vi "PCI-USB_ Untitled 1.vi"() -> ()   [LabVIEW 2015]
panel:
  in  "Output":T1={"DO"=FALSE, "DO 2"=FALSE, "DO 3"=FALSE, "DO 4"=FALSE, "DO 5"=FALSE, "DO 6"=FALSE, "DO 7"=FALSE, "DO 8"=FALSE, "DO 9"=FALSE, "DO 10"=FALSE, "DO 11"=FALSE, "DO 12"=FALSE, "DO 13"=FALSE, "DO 14"=FALSE, "DO 15"=FALSE, "DO 16"=FALSE, "Signal Name"="", "Signal Name 2"="", "Signal Name 3"="", "Signal Name 4"="", "Signal Name 5"="", "Signal Name 6"="", "Signal Name 7"="", "Signal Name 8"="", "Signal Name 9"="", "Signal Name 10"="", "Signal Name 11"="", "Signal Name 12"="", "Signal Name 13"="", "Signal Name 14"="", "Signal Name 15"="", "Signal Name 16"="", "S,N0"="0", "S,N0 2"="1", "S,N0 3"="2", "S,N0 4"="3", "S,N0 5"="4", "S,N0 6"="5", "S,N0 7"="6", "S,N0 8"="7", "S,N0 9"="8", "S,N0 10"="9", "S,N0 11"="10", "S,N0 12"="11", "S,N0 13"="12", "S,N0 14"="13", "S,N0 15"="14", "S,N0 16"="15"}
  out "Array Element.Label.Text":string
  out "Label.Text":string
  out "NewVal[8].DO":bool
  in  "stop":bool
  out "DO":bool
  in  "Digital Output":T2(array[cluster])=[{"DO"=FALSE, "Signal Name"="Rotating servo pulse", "S,N0"="0"}, {"DO"=FALSE, "Signal Name"="Oscilating servo pulse", "S,N0"="1"}, {"DO"=FALSE, "Signal Name"="Rotating servo direction", "S,N0"="2"}, {"DO"=FALSE, "Signal Name"="Oscilating servo direction", "S,N0"="3"}, {"DO"=FALSE, "Signal Name"="Both Servo fault", "S,N0"="4"}, {"DO"=FALSE, "Signal Name"="Unit slide cyl up sol.", "S,N0"="5"}, {"DO"=FALSE, "Signal Name"="Unit slide cyl dn sol.", "S,N0"="6"}, {"DO"=FALSE, "Signal Name"="Gripper close sol.", "S,N0"="7"}, {"DO"=FALSE, "Signal Name"="Clamping  Cyl Dn Sol.", "S,N0"="8"}, {"DO"=FALSE, "Signal Name"="Dot punching cyl fwd Sol.", "S,N0"="9"}, {"DO"=FALSE, "Signal Name"="Ok Indicator TWL/Green", "S,N0"="10"}, {"DO"=FALSE, "Signal Name"="Fault Indicator TWL/red buzzer", "S,N0"="11"}, {"DO"=FALSE, "Signal Name"="Running Indicator TWL/Yellow", "S,N0"="12"}, {"DO"=FALSE, "Signal Name"="SPARE", "S,N0"="13"}, {"DO"=FALSE, "Signal Name"="SPARE", "S,N0"="14"}, {"DO"=FALSE, "Signal Name"="SPARE", "S,N0"="15"}]
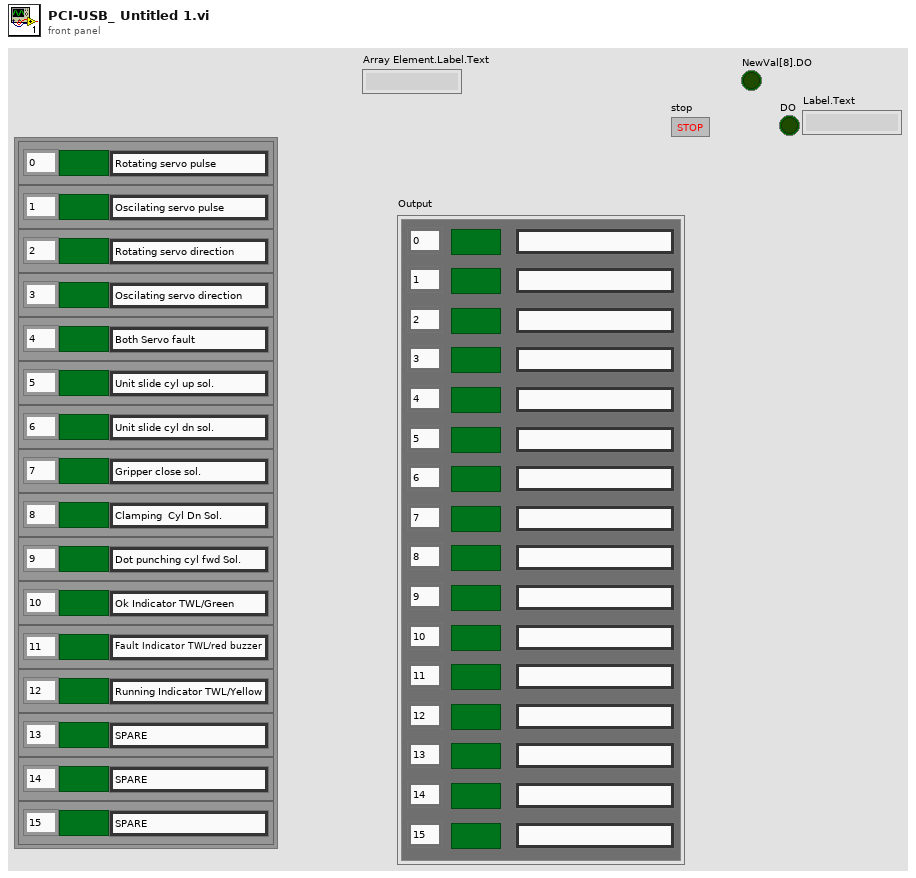
[diagram p1: front panel]
types:
  T1 = cluster{"DO":bool, "DO 2":bool, "DO 3":bool, "DO 4":bool, "DO 5":bool, "DO 6":bool, "DO 7":bool, "DO 8":bool, "DO 9":bool, "DO 10":bool, "DO 11":bool, "DO 12":bool, "DO 13":bool, "DO 14":bool, "DO 15":bool, "DO 16":bool, "Signal Name":string, "Signal Name 2":string, "Signal Name 3":string, "Signal Name 4":string, "Signal Name 5":string, "Signal Name 6":string, "Signal Name 7":string, "Signal Name 8":string, "Signal Name 9":string, "Signal Name 10":string, "Signal Name 11":string, "Signal Name 12":string, "Signal Name 13":string, "Signal Name 14":string, "Signal Name 15":string, "Signal Name 16":string, "S,N0":string, "S,N0 2":string, "S,N0 3":string, "S,N0 4":string, "S,N0 5":string, "S,N0 6":string, "S,N0 7":string, "S,N0 8":string, "S,N0 9":string, "S,N0 10":string, "S,N0 11":string, "S,N0 12":string, "S,N0 13":string, "S,N0 14":string, "S,N0 15":string, "S,N0 16":string}
  T2 = cluster{"DO":bool, "Signal Name":string, "S,N0":string}[]
  T3 = cluster{"NewVal[0]":cluster{"DO":bool, "Signal Name":string, "S,N0":string}, "NewVal[1]":cluster{"DO":bool, "Signal Name":string, "S,N0":string}, "NewVal[2]":cluster{"DO":bool, "Signal Name":string, "S,N0":string}, "NewVal[3]":cluster{"DO":bool, "Signal Name":string, "S,N0":string}, "NewVal[4]":cluster{"DO":bool, "Signal Name":string, "S,N0":string}, "NewVal[5]":cluster{"DO":bool, "Signal Name":string, "S,N0":string}, "NewVal[6]":cluster{"DO":bool, "Signal Name":string, "S,N0":string}, "NewVal[7]":cluster{"DO":bool, "Signal Name":string, "S,N0":string}, "NewVal[8]":cluster{"DO":bool, "Signal Name":string, "S,N0":string}, "NewVal[9]":cluster{"DO":bool, "Signal Name":string, "S,N0":string}, "NewVal[10]":cluster{"DO":bool, "Signal Name":string, "S,N0":string}, "NewVal[11]":cluster{"DO":bool, "Signal Name":string, "S,N0":string}, "NewVal[12]":cluster{"DO":bool, "Signal Name":string, "S,N0":string}, "NewVal[13]":cluster{"DO":bool, "Signal Name":string, "S,N0":string}, "NewVal[14]":cluster{"DO":bool, "Signal Name":string, "S,N0":string}, "NewVal[15]":cluster{"DO":bool, "Signal Name":string, "S,N0":string}}
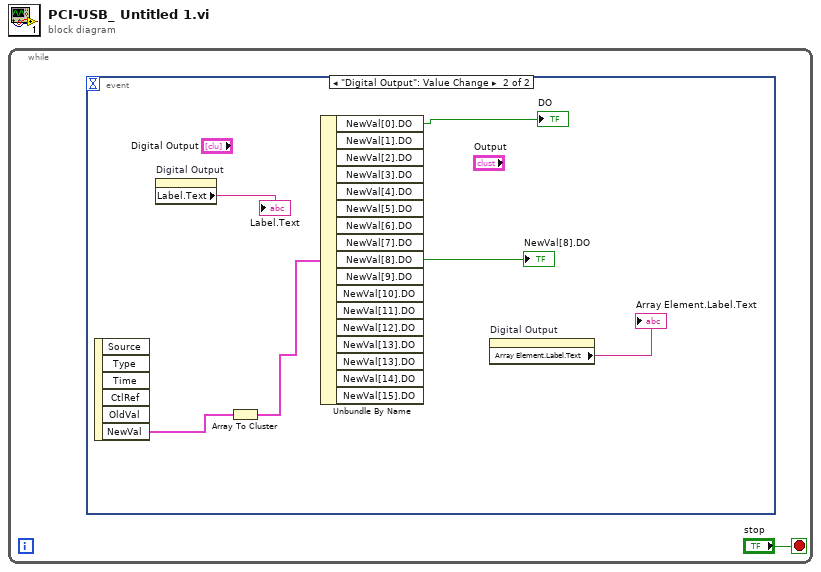
[diagram p0: block diagram]
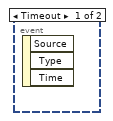
[diagram p2: hidden frame]
diagram:
  n1 = while {
    stop <- "stop" stop-if-true
    n2 = event shown="[1] \"Digital Output\": Value Change" {
      selector: _ -> [_ _]
      dyn-events: _ -> [_ _]
      timeout: _ -> [_ _]
      event Timeout {
        n3 = event-data() -> ()  [unwired: 1 in, 3 out]
      }
      event "Digital Output": Value Change {
        n4 = event-data() -> ("NewVal"=w4:T2)  [unwired: 1 in, 5 out]
        n5 = property on="Digital Output" class="Arr (strict)"() -> ("Label.Text"=→"Label.Text":string)  [unwired: 2 in, 2 out]
        n6 = Array To Cluster(array=w4) -> (cluster=w6:T3)
        n7 = Unbundle By Name(w6) -> ("NewVal[0].DO"=→"DO":bool, "NewVal[8].DO"=→"NewVal[8].DO":bool)  [unwired: 15 out]
        n8 = property on="Digital Output" class="Arr (strict)"() -> ("Array Element.Label.Text"=→"Array Element.Label.Text":string)  [unwired: 2 in, 2 out]
      }
    }
  }
